vi "test_Format Instrument String Command_Format array command(Padding Enabled).vi"(8 "error in (no error)":errorcluster, 11 "TestCase in":refnum<class "Instrument Addon Unit Tests.lvclass">) -> (0 "error out":errorcluster, 3 "TestCase out":refnum<class "Instrument Addon Unit Tests.lvclass">)   [LabVIEW 2019, in "Instrument Addon Unit Tests.lvclass"]
uses:
  Instrument Addon Unit Tests.lvclass
  Addon/Addon Shared/Types/Command Parameters.ctl
  Addon/Addon Shared/Types/Linked Channel Cluster.ctl
  Addon/Addon Shared/Types/Meta Data RT Configuration Cluster.ctl
  Addon/Addon Shared/Types/MetaData Parameters.ctl
  Addon/Addon Shared/Types/Protocol Data Type.ctl
  Addon/Addon Shared/Types/Metadata Channel Type.ctl
  Addon/Addon Shared/Types/Type Cast Type.ctl
  Addon/Addon Shared/Types/Endian.ctl
  Addon/Addon Engine/SubVIs/Format Numeric to String.vi
  <vilib>/addons/_JKI Toolkits/VI Tester/TestCase.llb/TestCase.lvclass
  Addon/Addon Engine/Instrument Addon Engine.lvlib
  Addon/Addon Shared/Instrument Addon Shared.lvlib
  C:/Program Files (x86)/National Instruments/LabVIEW 2019/vi.lib/addons/_JKI Toolkits/VI Tester/TestCase.llb/TestCase.lvclass
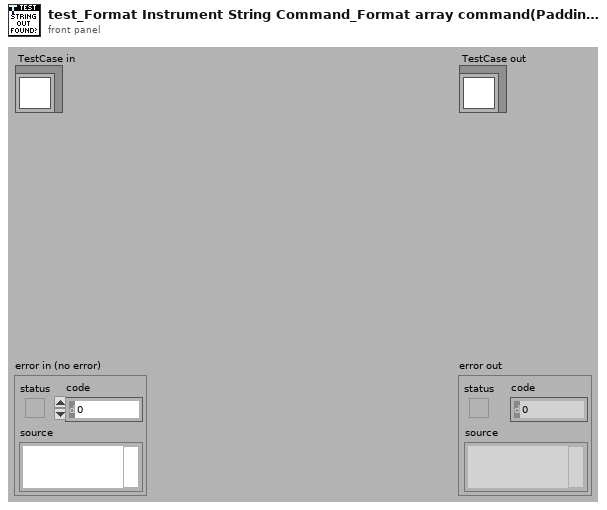
[diagram p1: front panel]
types:
  T1 = typedef "Instrument Addon Shared.lvlib/Meta Data RT Configuration Cluster.ctl" = cluster{"MetaData Parameters":T2, "Data Index":i32, "Data Length":i32}
  T2 = typedef "Instrument Addon Shared.lvlib/MetaData Parameters.ctl" = cluster{"Data Type":T3, "Channel Type":T4, "List":string[], "Format String":string, "Type":T5, "Delimiter":string, "Endian":T6}
  T3 = typedef "Instrument Addon Shared.lvlib/Protocol Data Type.ctl" = enum16{"Single Channel", "Array"}
  T4 = typedef "Instrument Addon Shared.lvlib/Metadata Channel Type.ctl" = enum16{"Enumerated List", "Format", "Type Cast"}
  T5 = typedef "Instrument Addon Shared.lvlib/Type Cast Type.ctl" = enum16{"DBL", "SGL", "U64", "U32", "U16", "U8", "I64", "I32", "I16", "I8"}
  T6 = typedef "Instrument Addon Shared.lvlib/Endian.ctl" = enum16{"Native", "Little", "Big"}
  T7 = typedef "Instrument Addon Shared.lvlib/Command Parameters.ctl" = cluster{"Command":string, "Linked Channels":T8[], "Pad":bool, "Length":u32, "Pad Value":u8}
  T8 = typedef "Instrument Addon Shared.lvlib/Linked Channel Cluster.ctl" = cluster{"Variable Name":string, "GUID":string}
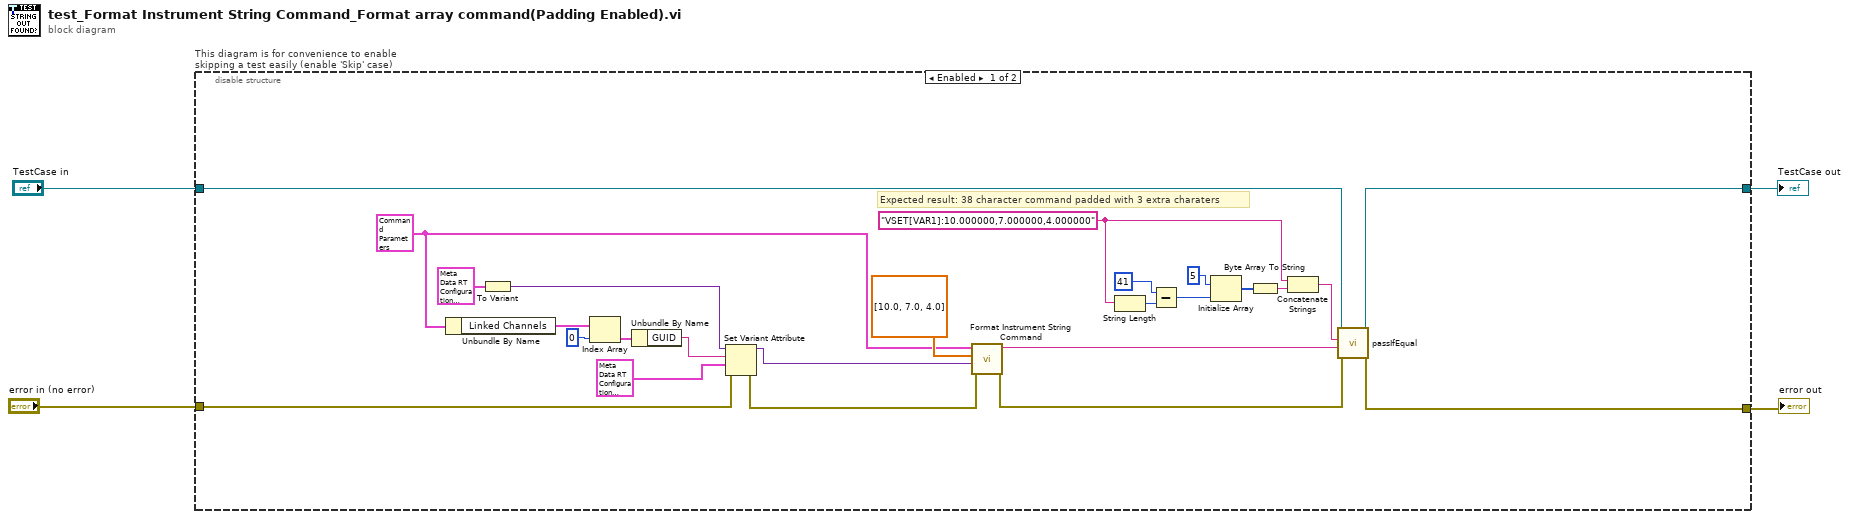
[diagram p0: block diagram]
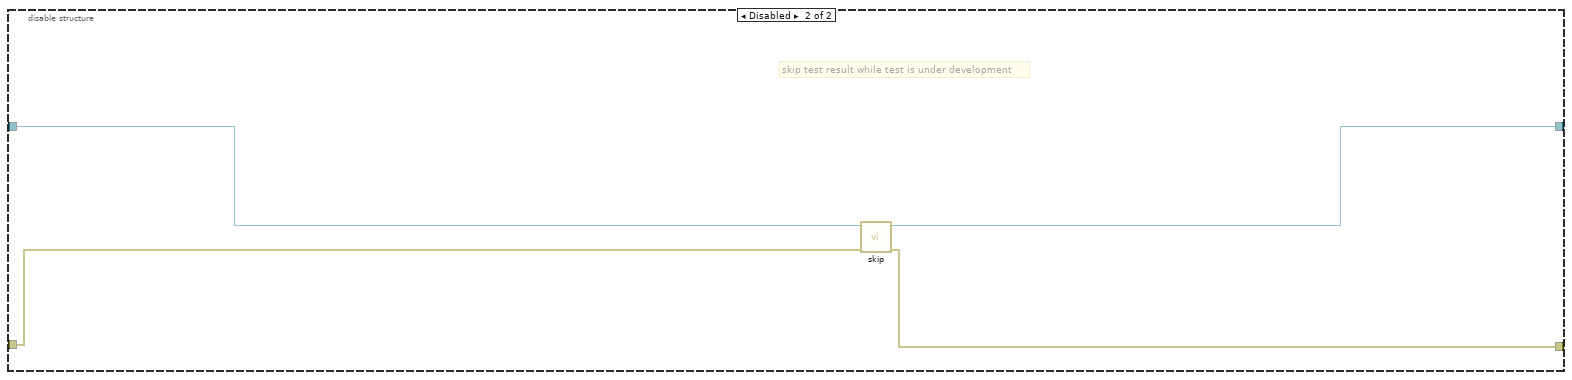
[diagram p2: hidden frame]
diagram:
  n1 = disable-structure "This diagram is for convenience to enable skipping a test easily (enable 'Skip' case)" shown="Enabled" {
    disable-tunnel: "TestCase in" -> [w29 w33]
    disable-tunnel: [w14 w31] -> w1
    disable-tunnel: [w28 w32] -> w3
    disable-tunnel: "error in (no error)" -> [w16 w30]
    frame Enabled {
      w9 = "VSET[VAR1]:10.000000,7.000000,4.000000" ("Command")
      w22 = T7 {"Command"="VSET[VAR1]:[MetadataChannel]", "Linked Channels"=[{"Variable Name"="MetadataChannel", "GUID"="9428600d-6a85-43b8-aaac-a755da7e0c9b"}], "Pad"=TRUE, "Length"=41, "Pad Value"=5} ("Command Parameters")
      # "Expected result: 38 character command padded with 3 extra charaters"
      n2 = Unbundle By Name(w22) -> ("Linked Channels"=w21:T8[])
      n3 = To Variant(anything=T1 {"MetaData Parameters"={"Data Type"=enum."Single Channel", "Channel Type"=enum."Enumerated List", "List"=[], "Format String"="", "Type"=enum."DBL", "Delimiter"="", "Endian"=enum."Native"}, "Data Index"=0, "Data Length"=0}) -> (Variant=w25:variant)
      n4 = Index Array(array=w21, index=0) -> (element=w19:T8)
      n5 = Unbundle By Name(w19) -> ("GUID"=w18:string)
      n6 = Set Variant Attribute(Variant=w25, name=w18, value=T1 {"MetaData Parameters"={"Data Type"=enum."Array", "Channel Type"=enum."Format", "List"=[], "Format String"="", "Type"=enum."DBL", "Delimiter"=",", "Endian"=enum."Native"}, "Data Index"=0, "Data Length"=3}, error in=w16) -> (Variant out=w24:variant, error out=w15:errorcluster)  [unwired: 1 out]
      n7 = call "Format Instrument String Command.vi"("error in (no error)"=w15, "MetaData Lookup in"=w24, "MetaData"=dbl[] [10.0, 7.0, 4.0], "Command Parameters"=w22) -> ("error out"=w27:errorcluster, "Command"=w13:string)  [unwired: 5 in, 1 out]
      n8 = String Length(string=w9) -> (length=w12:i32)
      n9 = Subtract(x=41, y=w12) -> (x-y=w11:i32)
      n10 = Initialize Array(u8 5 ("element"), w11) -> (w5:u8[])
      n11 = Byte Array To String(unsigned byte array=w5) -> (string=w10:string)
      n12 = Concatenate Strings(w9, w10) -> (w6:string)
      n13 = call-dynamic "passIfEqual.vi"("error in (no error)"=w27, "y"=w13, "x"=w6, "TestCase in"=w29) -> ("error out"=w28:errorcluster, "TestCase out"=w14:refnum<class "Instrument Addon Unit Tests.lvclass">)  [unwired: 6 in]
    }
    frame Disabled {
      # "skip test result while test is under development"
      n14 = call <vilib>:"skip.vi"("error in (no error)"=w30, "TestCase in"=w33) -> ("error out"=w32:errorcluster, "TestCase out"=w31:refnum<class "Instrument Addon Unit Tests.lvclass">)  [unwired: 8 in]
    }
  }
  "error out" <- w3
  "TestCase out" <- w1
